vi "Linear Programming Preparation.vi"(4 "dim2(M)":i32, 5 "dim1 (M)":i32, 6 "M":dbl[][](array[numeric]) format="%.2f", 7 "B":dbl[](array[numeric]) format="%.2f") -> (0 "dim1+dim2":i32, 1 "n-m":u32[](array[numeric]), 2 "m":u32[](array[numeric]), 3 "Table":dbl[][](array[numeric]) format="%.2f")   [LabVIEW 2020, in "NI_Gmath.lvlib"]
uses:
  NI_Gmath.lvlib
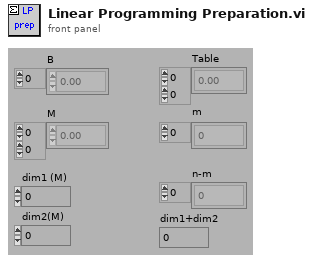
[diagram p1: front panel]
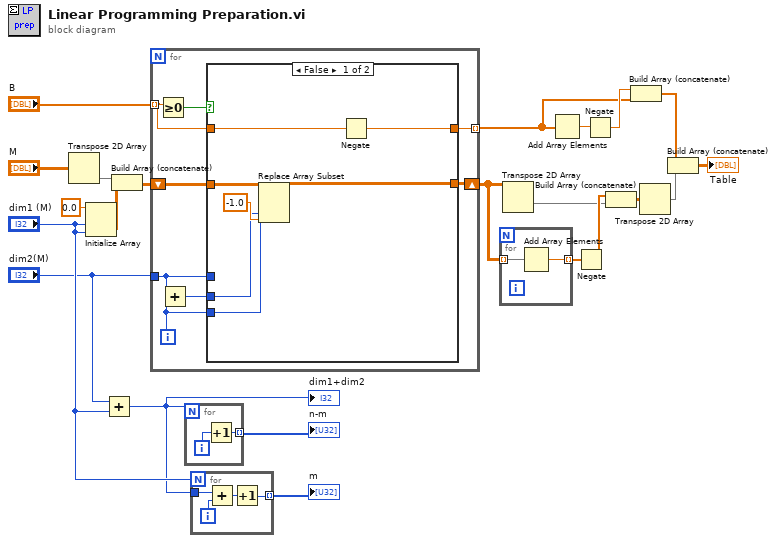
[diagram p0: block diagram]
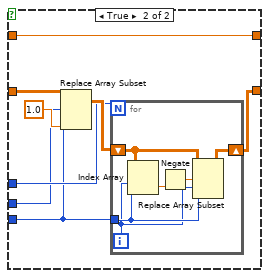
[diagram p2: hidden frame]
diagram:
  n1 = Transpose 2D Array(2D array="M") -> (transposed array=w19:dbl[][])
  n2 = Initialize Array(0.0, "dim1 (M)", "dim1 (M)") -> (w20:dbl[][])
  n3 = Add(x="dim2(M)", y="dim1 (M)") -> (x+y=w1:i32)
  "dim1+dim2" <- w1
  n4 = Build Array (concatenate)(w19, w20) -> (w16:dbl[][])
  n5 = for {
    tunnel: "B" -> [w24] mode=indexing
    tunnel: "dim2(M)" -> [w25]
    shift-right: [w26] -> w2
    shift-left: w16 -> [w27]
    tunnel: [w23] -> w12 mode=indexing
    i -> [w28]
    n6 = Greater Or Equal To 0?(x=w24) -> (x >= 0?=w30:bool)
    n7 = Add(x=w25, y=w28) -> (x+y=w29:i32)
    n8 = case shown="False" w30 {
      tunnel: w29 -> [w32 w40]
      tunnel: w28 -> [w33 w39]
      tunnel: w27 -> [w36 w44]
      tunnel: [w35 w42] -> w26
      tunnel: w25 -> [_ w41]
      tunnel: w24 -> [w34 w38]
      tunnel: [w31 w38] -> w23
      frame False {
        n9 = Replace Array Subset(array=w36, new element=-1.0, index (row)=w32, index (col)=w33) -> (w35:dbl[][])
        n10 = Negate(x=w34) -> (-x=w31:dbl)
      }
      frame True {
        n11 = Replace Array Subset(array=w44, new element=1.0, index (row)=w40, index (col)=w39) -> (w43:dbl[][])
        n12 = for {
          N: w41 -> [_]
          shift-right: [w51] -> w42
          shift-left: w43 -> [w50]
          tunnel: w39 -> [w47]
          i -> [w46]
          n13 = Index Array(array=w50, index (row)=w46, index (col)=w47) -> (element=w49:dbl)
          n14 = Negate(x=w49) -> (-x=w48:dbl)
          n15 = Replace Array Subset(array=w50, new element=w48, index (row)=w46, index (col)=w47) -> (w51:dbl[][])
        }
      }
    }
  }
  n16 = for {
    N: w1 -> [_]
    tunnel: [w52] -> w14 mode=indexing
    i -> [w53]
    n17 = Increment(x=w53) -> (x+1=w52:i32)
  }
  "n-m" <- w14
  n18 = for {
    N: "dim1 (M)" -> [_]
    tunnel: w1 -> [w57]
    tunnel: [w54] -> w3 mode=indexing
    i -> [w56]
    n19 = Add(x=w57, y=w56) -> (x+y=w55:i32)
    n20 = Increment(x=w55) -> (x+1=w54:i32)
  }
  "m" <- w3
  n21 = for {
    tunnel: w2 -> [w59] mode=indexing
    tunnel: [w58] -> w17 mode=indexing
    n22 = Add Array Elements(numeric array=w59) -> (sum=w58:dbl)
  }
  n23 = Transpose 2D Array(2D array=w2) -> (transposed array=w8:dbl[][])
  n24 = Add Array Elements(numeric array=w12) -> (sum=w15:dbl)
  n25 = Negate(x=w17) -> (-x=w11:dbl[])
  n26 = Negate(x=w15) -> (-x=w13:dbl)
  n27 = Build Array (concatenate)(w11, w8) -> (w7:dbl[][])
  n28 = Build Array (concatenate)(w13, w12) -> (w10:dbl[])
  n29 = Transpose 2D Array(2D array=w7) -> (transposed array=w6:dbl[][])
  n30 = Build Array (concatenate)(w10, w6) -> (→"Table":dbl[][])
